vi "Stop Autostop Nested Actors_Stops Nested Actors.vi"() -> ()   [LabVIEW 2020]
uses:
  Test Harness/Actor with Nesteds/Actor with Nesteds/Actor with Nesteds.lvclass
  ActorFramework/Actor/Actor.lvclass
  ActorFramework/Message Queue/Message Queue.lvclass
  Test Harness/Actor with Nesteds/Actor with Nesteds Messages/Stop Nested Actors Msg/Stop Nested Actors Msg.lvclass
  ActorFramework/Message Dequeuer/Message Dequeuer.lvclass
  <vilib>/addons/_JKI Toolkits/Caraya/classes/Assert/Assert Equal Value_Variant.vi
  ActorFramework/Stop Msg/Stop Msg.lvclass
  C:/Users/Neil/Documents/actor-framework/Core/ActorFramework/Actor/Actor.lvclass
  C:/Users/Neil/Documents/actor-framework/Core/Testing/Test Harness/Actor with Nesteds/Actor with Nesteds/Actor with Nesteds.lvclass
panel:
  out "error out":errorcluster
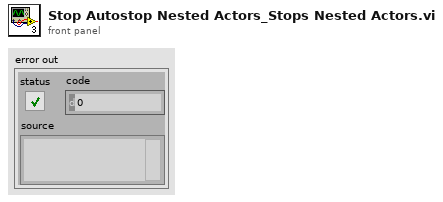
[diagram p1: front panel]
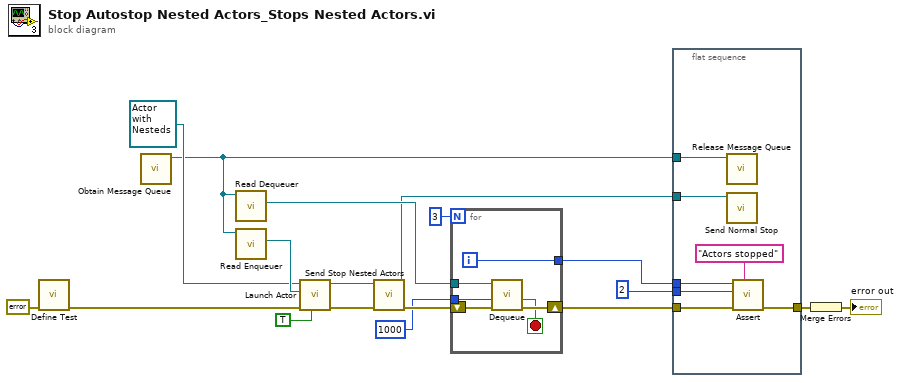
[diagram p0: block diagram]
diagram:
  n1 = call <vilib>:"Define Test.vi"("error in (no error)"=errorcluster {"status"=FALSE, "code"=0, "source"=""}) -> ("error out"=w16:errorcluster)  [unwired: 9 in, 1 out]
  n2 = call "Obtain Message Queue.vi"() -> ("Message Queue"=w6:refnum<class "Message Queue.lvclass">)  [unwired: 10 in, 1 out]
  n3 = call "Read Dequeuer.vi"("Message Queue"=w6) -> ("Message Dequeuer"=w10:refnum<class "Message Dequeuer.lvclass">)  [unwired: 10 in]
  n4 = call "Read Enqueuer.vi"("Message Queue"=w6) -> ("Message Enqueuer"=w15:refnum<class "Message Enqueuer.lvclass">)  [unwired: 10 in]
  n5 = call "Launch Actor.vi"("Open Actor Core front panel? (F)"=TRUE, "error in (no error)"=w16, "Actor-to-Caller Enqueuer"=w15, "Actor"=refnum<class "Actor with Nesteds.lvclass"> refnum ("Actor with Nesteds.lvlib:Actor with Nesteds.lvclass")) -> ("error out"=w14:errorcluster, "Caller-To-Actor Enqueuer"=w13:refnum<class "Message Enqueuer.lvclass">)  [unwired: 6 in]
  n6 = call "Send Stop Nested Actors.vi"("error in (no error)"=w14, "Message Enqueuer"=w13) -> ("error out"=w12:errorcluster, "Message Enqueuer out"=w1:refnum<class "Message Enqueuer.lvclass">)  [unwired: 8 in]
  n7 = for {
    N: 3 -> [_]
    tunnel: u32 1000 ("milliseconds to wait") -> [w23]
    tunnel: w10 -> [w22]
    shift-right: [w21] -> w9
    shift-left: w12 -> [w24]
    tunnel: [w19] -> w3
    i -> [w19]
    stop <- w20 stop-if-true
    n8 = call "Dequeue.vi"("error in (no error)"=w24, "timeout in ms (-1)"=w23, "Message Dequeuer in"=w22) -> ("error out"=w21:errorcluster, "timed out?"=w20:bool)  [unwired: 4 in, 3 out]
  }
  n9 = flat-sequence {
    tunnel: [w30] -> w18
    tunnel: w9 -> [w29]
    tunnel: w6 -> [w28]
    tunnel: w3 -> [w27]
    tunnel: 2 -> [w26]
    tunnel: w1 -> [w25]
    frame #0 {
      n10 = call "Release Message Queue.vi"("Message Queue"=w28) -> ()  [unwired: 9 in, 2 out]
      n11 = call "Send Normal Stop.vi"("Message Enqueuer"=w25) -> ()  [unwired: 10 in, 1 out]
      n12 = call-poly <vilib>:"Assert.vi"("Label"="Actors stopped" ("Label (VI Title)"), "error in (no error)"=w29, "Y"=w26, "X"=w27) -> ("error out"=w30:errorcluster)  [unwired: 6 in, 1 out]
    }
  }
  n13 = Merge Errors(w18) -> (→"error out":errorcluster)
